vi "LeftButtonDown.vi"(8 "Error in (no error)":errorcluster, 11 "Click?":bool=TRUE) -> (0 "Error out":errorcluster)   [LabVIEW 2013]
uses:
  user32.dll
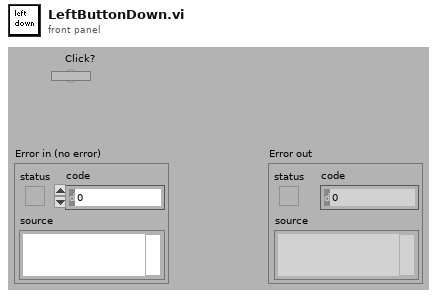
[diagram p1: front panel]
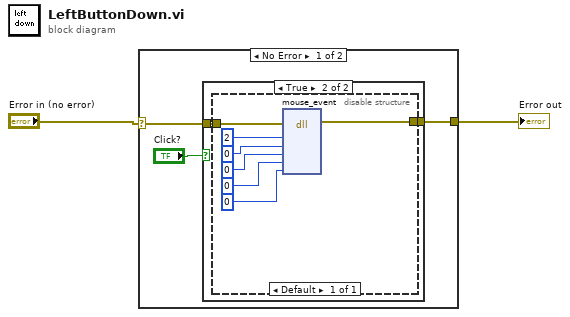
[diagram p0: block diagram]
diagram:
  n1 = case shown="No Error" "Error in (no error)" {
    selector: "Error in (no error)" -> [w5 w16]
    tunnel: [w4 w16] -> w1
    frame No Error {
      n2 = case shown="True" "Click?" {
        tunnel: w5 -> [w6 w8]
        tunnel: [w6 w7] -> w4
        frame False {
        }
        frame True {
          n3 = disable-structure shown="Default" {
            disable-tunnel: w8 -> [w10]
            disable-tunnel: [w9] -> w7
            frame Enabled {
              n4 = dll-call lib="user32.*" fn="mouse_event"(error in=w10, "dwFlags"=u32 2, "dx"=u32 0, "dy"=u32 0, "dwData"=u32 0, "dxExtraInfo"=u32 0) -> (error out=w9:errorcluster)  [unwired: 7 in, 2 out]
            }
          }
        }
      }
    }
    frame Error {
    }
  }
  "Error out" <- w1
